vi "Sliding Menu Facade.vi"(0 "Data In":T5, 2 "Display State In":T2={"Numeric"=0.0, "Array of Button References"=[], "Space Between Menu Buttons"=0, "Number of Menu Buttons"=0, "Array of Button Names"=[], "Most Recent Vertical Position"=0, "This VI"=refnum, "Current Action"=enum."Not Moving", "Most Recent Distance Traveled"=0, "Method"=enum."Move Up", "Data In"=0}, 3 "Container State":T6) -> (6 "Data Out":T5, 7 "Display State Out":T2={"Numeric"=0.0, "Array of Button References"=[], "Space Between Menu Buttons"=0, "Number of Menu Buttons"=0, "Array of Button Names"=[], "Most Recent Vertical Position"=0, "This VI"=refnum, "Current Action"=enum."Not Moving", "Most Recent Distance Traveled"=0, "Method"=enum."Move Up", "Data In"=0}, 8 "Action":T1)   [LabVIEW 2011, in "Sliding Menu Library.lvlib" / "Sliding Menu XControl.xctl"]
uses:
  Sliding Menu XControl.xctl
  Sliding Menu Data.ctl
  <vilib>/_xctls/Container State.ctl
  Sliding Menu State.ctl
  Menu Button Library/Menu Button xControl/Menu Button xControl.xctl
  Sliding Menu SubVIs/Sliding Menu Type Definitions/Current User Action.ctl
  Sliding Menu Methods.ctl
  <vilib>/_xctls/Action.ctl
  <vilib>/_xctls/XControlSupport.lvlib
  Sliding Menu Library.lvlib
panel:
  in  "Button 7":bool(xcontrol)
  in  "Button 6":bool(xcontrol)
  in  "Button 5":bool(xcontrol)
  in  "Button 4":bool(xcontrol)
  in  "Button 3":bool(xcontrol)
  in  "Button 2":bool(xcontrol)
  in  "Button 1":bool(xcontrol)
  in  "Button 0":bool(xcontrol)
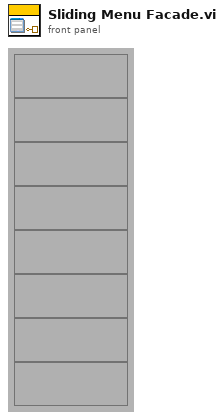
[diagram p1: front panel]
types:
  T1 = typedef "XControlSupport.lvlib/Action.ctl" = cluster{"Data Changed?":bool, "State Changed?":bool, "Action Name":string}
  T2 = typedef "Sliding Menu Library.lvlib/Sliding Menu XControl.xctl/Sliding Menu State.ctl" = cluster{"Numeric":dbl, "Array of Button References":refnum<vi>[], "Space Between Menu Buttons":i32, "Number of Menu Buttons":i32, "Array of Button Names":string[], "Most Recent Vertical Position":i32, "This VI":refnum<vi>, "Current Action":T3, "Most Recent Distance Traveled":i32, "Method":T4, "Data In":T5}
  T3 = typedef "Sliding Menu Library.lvlib/Current User Action.ctl" = enum16{"Not Moving", "Mouse Down", "Mouse Up No Dragging", "Bounce Up Needed", "Bounce Down Needed", "Dragging", "Easing"}
  T4 = typedef "Sliding Menu Methods.ctl" = enum16{"Resize", "Move Up", "Move Down", "Move to 0"}
  T5 = typedef "Sliding Menu Library.lvlib/Sliding Menu XControl.xctl/Sliding Menu Data.ctl" = i32
  T6 = typedef "XControlSupport.lvlib/Container State.ctl" = cluster{"Indicator?":bool, "Run Mode?":bool, " Refnum":refnum<vi>}
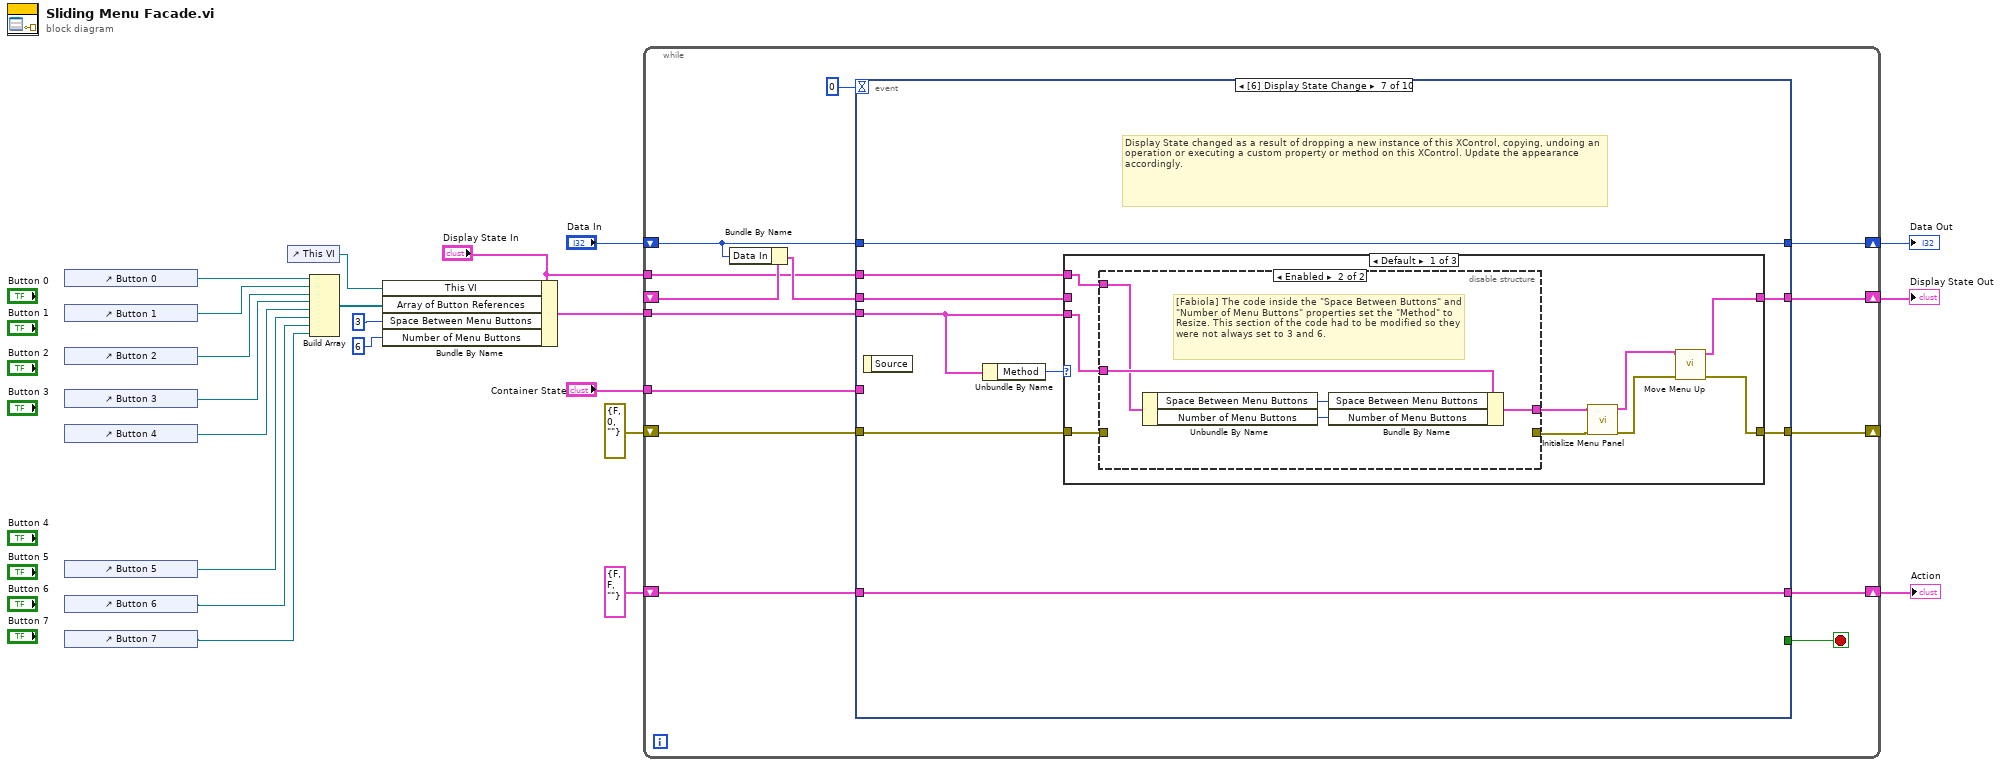
[diagram p0: block diagram]
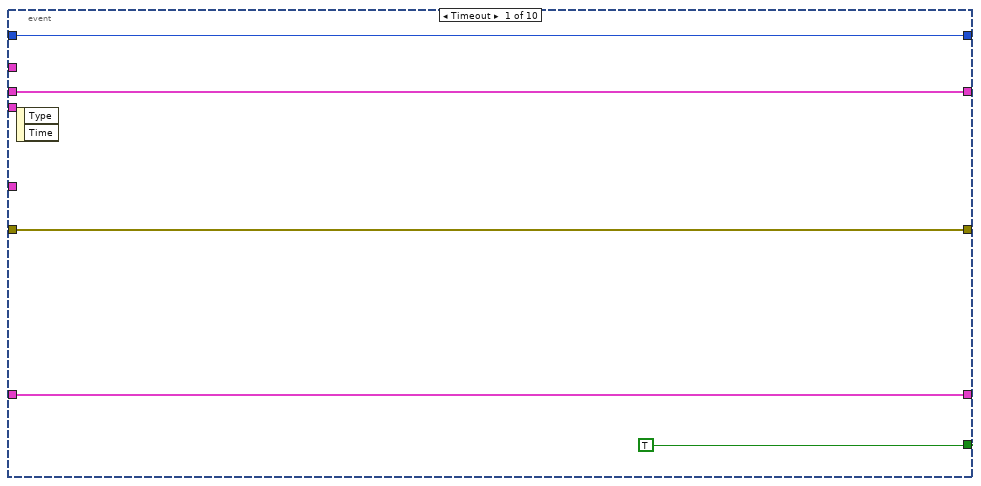
[diagram p2: hidden frame]
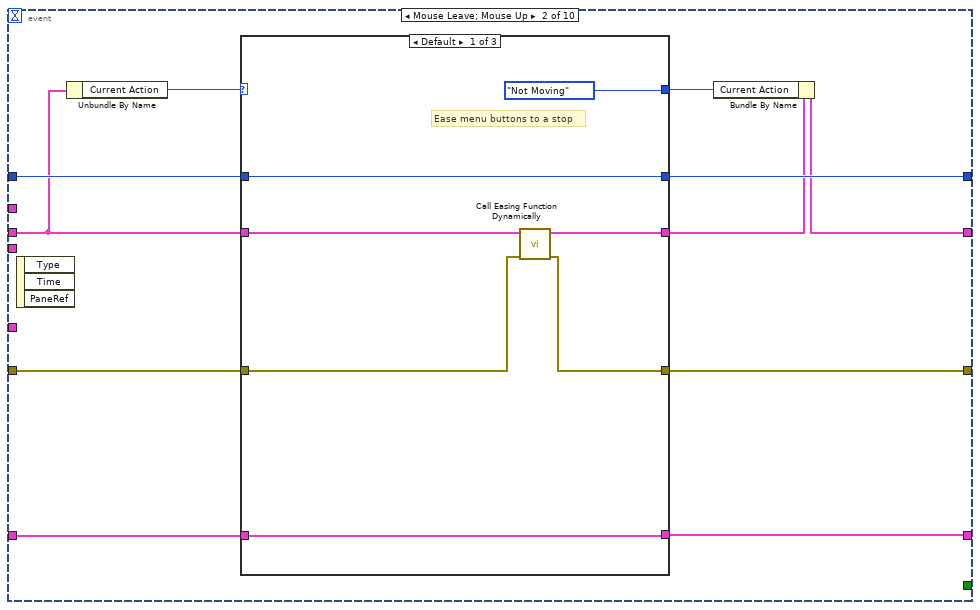
[diagram p3: hidden frame]
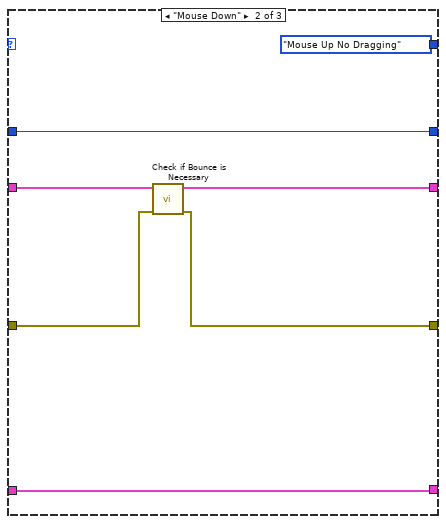
[diagram p4: hidden frame]
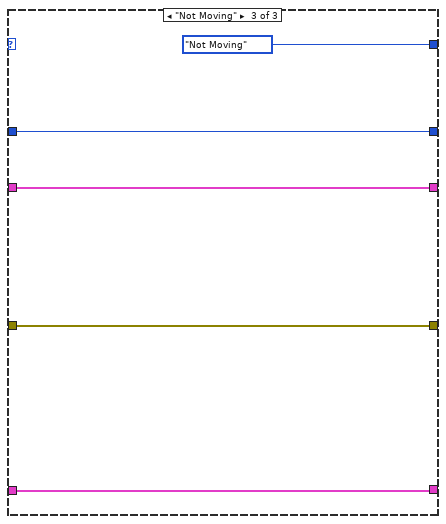
[diagram p5: hidden frame]
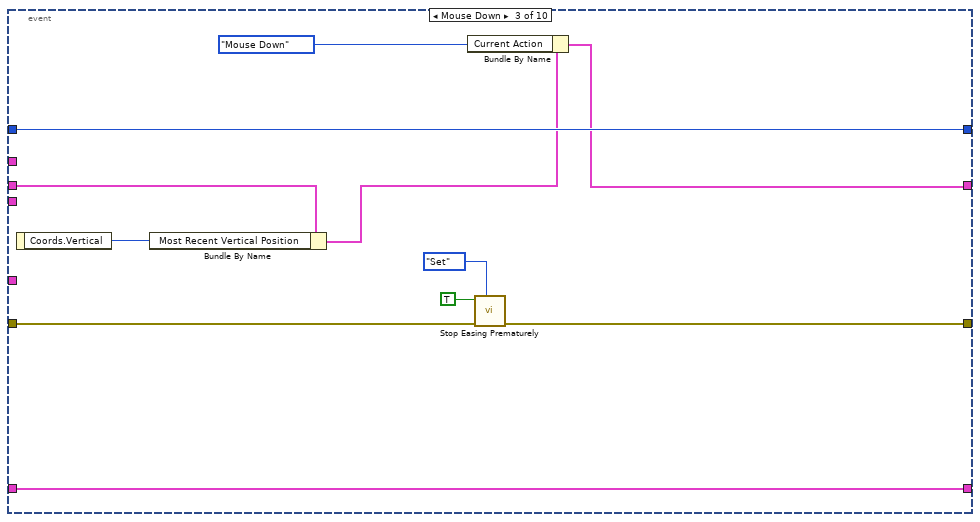
[diagram p6: hidden frame]
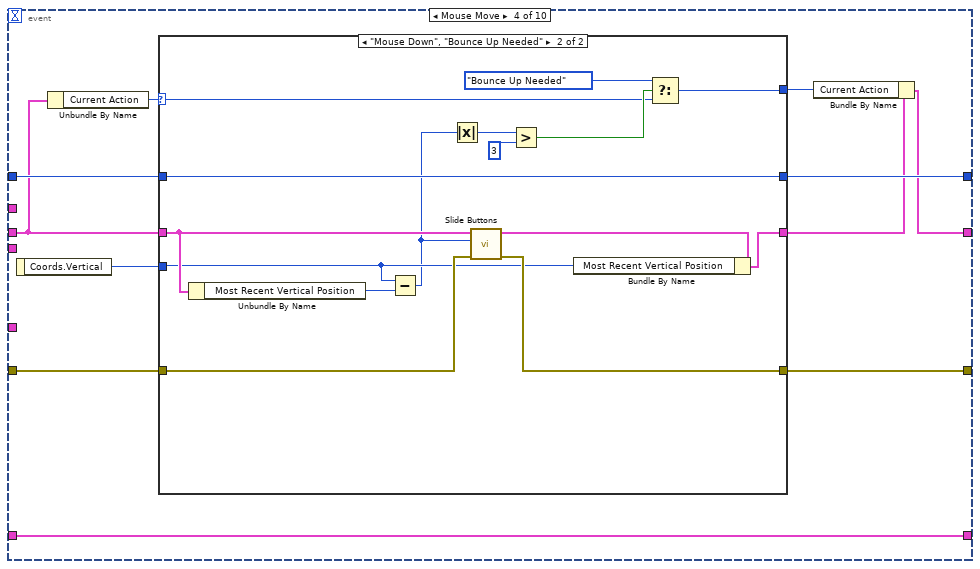
[diagram p7: hidden frame]
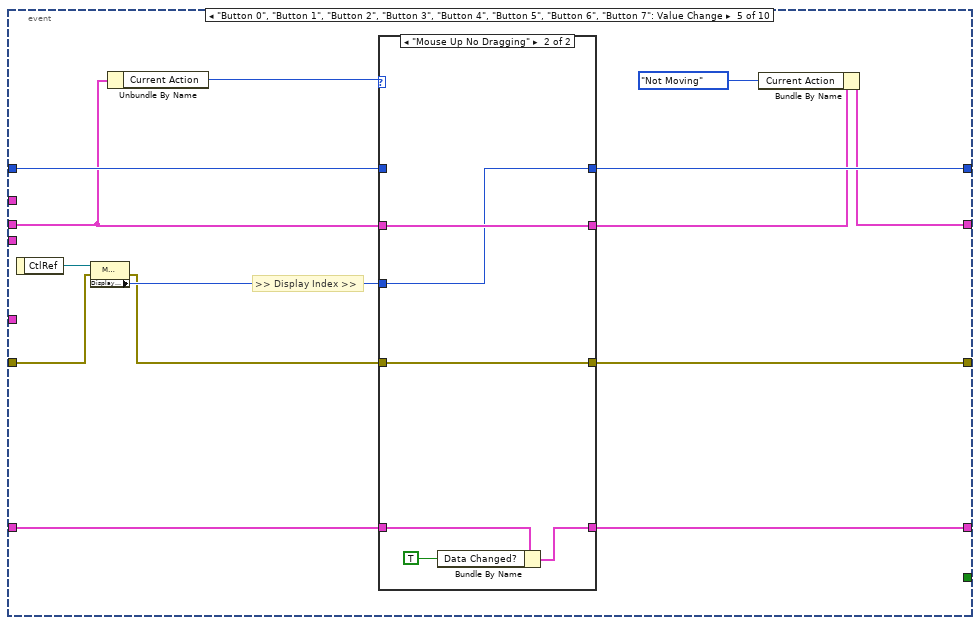
[diagram p9: hidden frame]
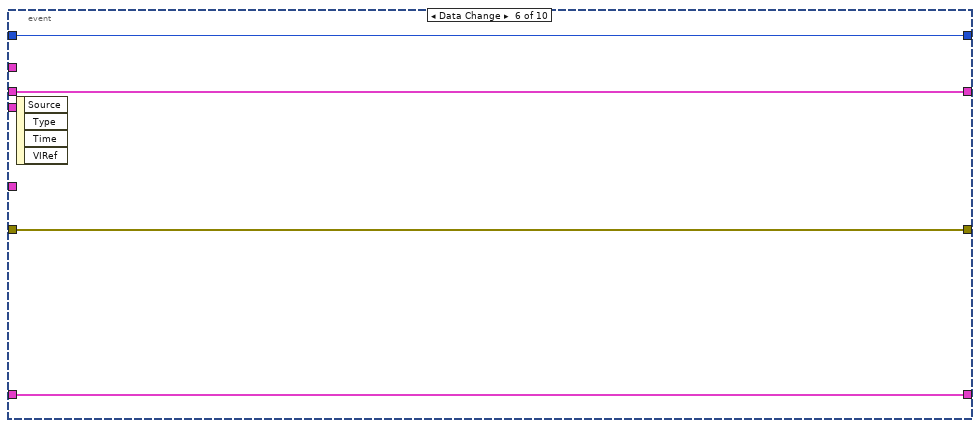
[diagram p11: hidden frame]
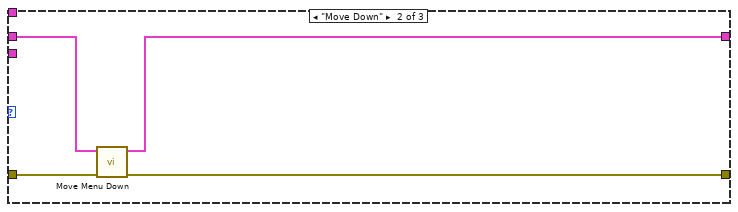
[diagram p13: hidden frame]
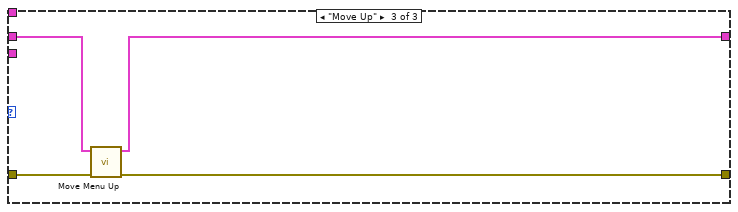
[diagram p14: hidden frame]
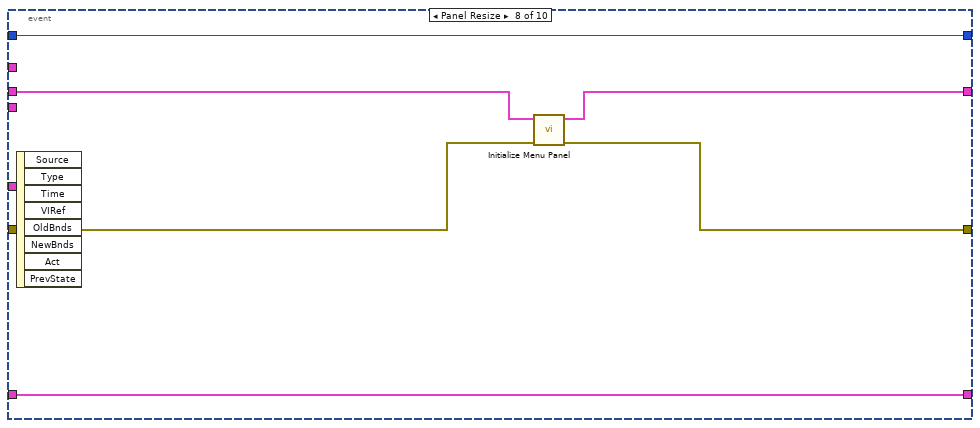
[diagram p15: hidden frame]
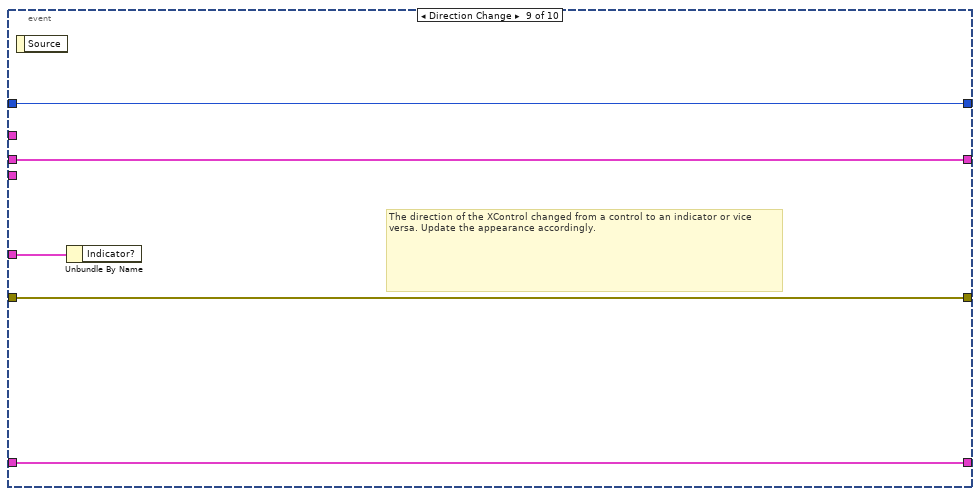
[diagram p16: hidden frame]
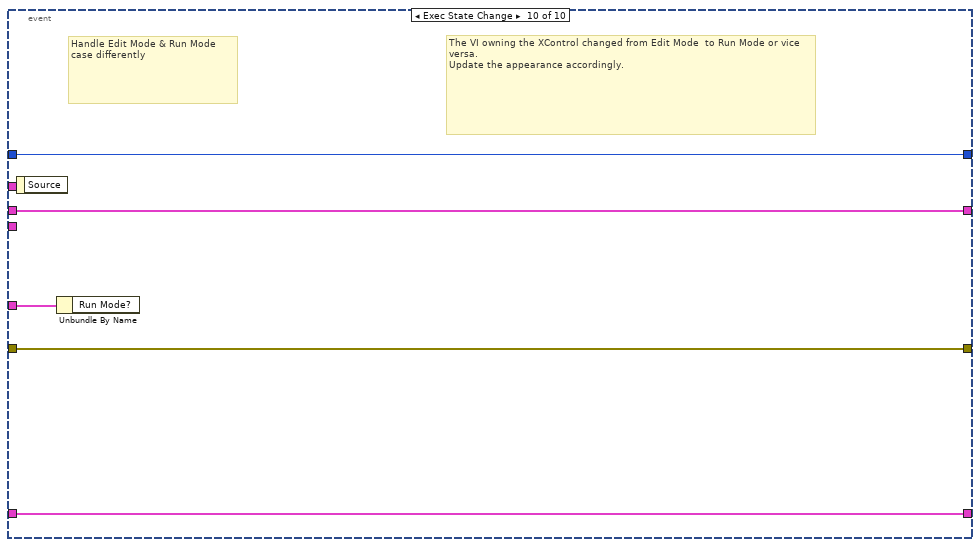
[diagram p17: hidden frame]
diagram:
  n1 = control-ref of="Button 0"() -> (w14:refnum<vi>)
  n2 = control-ref of="Button 1"() -> (w7:refnum<vi>)
  n3 = control-ref of="Button 2"() -> (w8:refnum<vi>)
  n4 = control-ref of="Button 3"() -> (w9:refnum<vi>)
  n5 = control-ref of="Button 4"() -> (w10:refnum<vi>)
  n6 = control-ref of="Button 5"() -> (w11:refnum<vi>)
  n7 = control-ref of="Button 6"() -> (w12:refnum<vi>)
  n8 = control-ref of="Button 7"() -> (w13:refnum<vi>)
  n9 = control-ref of="This VI"() -> (w5:refnum<vi>)
  n10 = Build Array(w14, w7, w8, w9, w10, w11, w12, w13) -> (w6:refnum<vi>[])
  n11 = Bundle By Name(cluster="Display State In", "This VI"=w5, "Array of Button References"=w6, "Space Between Menu Buttons"=3, "Number of Menu Buttons"=6) -> (w4:T2)
  n12 = while {
    shift-right: [w35] -> w19
    shift-left: _ -> [w25]
    tunnel: "Container State" -> [w32]
    shift-right: [w31] -> w21
    shift-left: "Data In" -> [w23]
    shift-right: [w29] -> w18
    shift-left: T1 {"Data Changed?"=FALSE, "State Changed?"=FALSE, "Action Name"=""} ("Action") -> [w30]
    shift-right: [w28] -> _
    shift-left: errorcluster {"status"=FALSE, "code"=0, "source"=""} ("error out") -> [w27]
    tunnel: w4 -> [w26]
    tunnel: "Display State In" -> [w22]
    stop <- w34 stop-if-true
    n13 = Bundle By Name(cluster=w25, "Data In"=w23) -> (w24:T2)
    n14 = event shown="[6] Display State Change" {
      selector: _ -> [_ _ _ _ _ _ _ _ _ _]
      dyn-events: _ -> [_ _ _ _ _ _ _ _ _ _]
      timeout: 0 -> [_ _ _ _ _ _ _ _ _ _]
      tunnel: w24 -> [w38 w45 w79 w86 w115 w138 w141 w176 w182 w187]
      tunnel: [w38 w42 w76 w83 w117 w138 w143 w175 w182 w187] -> w35
      tunnel: [TRUE _ _ _ _ _ _ _ _ _] -> w34
      tunnel: w32 -> [_ _ _ _ _ _ _ _ w183 w188]
      tunnel: w23 -> [w37 w48 w81 w90 w124 w139 w148 w178 w181 w186]
      tunnel: [w37 w49 w81 w91 w125 w139 w148 w178 w181 w186] -> w31
      tunnel: [w39 w46 w80 w92 w112 w137 w147 w177 w180 w185] -> w29
      tunnel: w30 -> [w39 w47 w80 w92 w113 w137 w147 w177 w180 w185]
      tunnel: [w36 w51 w71 w89 w123 w136 w145 w173 w179 w184] -> w28
      tunnel: w27 -> [w36 w50 w72 w88 w120 w136 w146 w174 w179 w184]
      tunnel: w26 -> [_ _ _ _ _ _ w144 _ _ _]
      tunnel: w22 -> [_ _ _ _ _ _ w140 _ _ _]
      event Timeout {
        n15 = event-data() -> ()  [unwired: 1 in, 2 out]
      }
      event Mouse Leave; Mouse Up {
        n16 = event-data() -> ()  [unwired: 1 in, 3 out]
        n17 = Unbundle By Name(w45) -> ("Current Action"=w44:T3)
        n18 = case shown="Default" w44 {
          tunnel: [Current_User_Action."Not Moving" ("Current Action") Current_User_Action."Mouse Up No Dragging" ("Current Action") Current_User_Action."Not Moving" ("Current Action")] -> w41
          tunnel: [w52 w59 w70] -> w51
          tunnel: w50 -> [w55 w60 w70]
          tunnel: [w57 w64 w69] -> w49
          tunnel: w48 -> [w57 w64 w69]
          tunnel: [w53 w61 w68] -> w43
          tunnel: w45 -> [w54 w62 w68]
          tunnel: [w56 w63 w67] -> w46
          tunnel: w47 -> [w56 w63 w67]
          frame Default {
            # "Ease menu buttons to a stop"
            n19 = call "Call Easing Function Dynamically.vi"("error in"=w55, "Display State In"=w54) -> ("error out"=w52:errorcluster, "Display State Out"=w53:T2)  [unwired: 8 in]
          }
          frame "Mouse Down" {
            n20 = call "Check if Bounce is Necessary.vi"("error in"=w60, "Display State In"=w62) -> ("error out"=w59:errorcluster, "Display State Out 2"=w61:T2)  [unwired: 7 in, 1 out]
          }
          frame "Not Moving" {
          }
        }
        n21 = Bundle By Name(cluster=w43, "Current Action"=w41) -> (w42:T2)
      }
      event Mouse Down {
        n22 = event-data() -> ("Coords.Vertical"=w78:i32)  [unwired: 1 in]
        n23 = Bundle By Name(cluster=w79, "Most Recent Vertical Position"=w78) -> (w75:T2)
        n24 = Bundle By Name(cluster=w75, "Current Action"=Current_User_Action."Mouse Down") -> (w76:T2)
        n25 = call "Stop Easing Prematurely.vi"("Set or Get Value"=enum16{"Set", "Get"}."Set", "error in"=w72, "Stop?"=TRUE) -> ("error out"=w71:errorcluster)  [unwired: 7 in, 1 out]
      }
      event Mouse Move {
        n26 = event-data() -> ("Coords.Vertical"=w87:i32)  [unwired: 1 in]
        n27 = Unbundle By Name(w86) -> ("Current Action"=w85:T3)
        n28 = case shown="\"Mouse Down\", \"Bounce Up Needed\"" w85 {
          selector: w85 -> [w93 w99]
          tunnel: [w93 w98] -> w82
          tunnel: [w94 w111] -> w91
          tunnel: w90 -> [w94 w111]
          tunnel: [w95 w104] -> w84
          tunnel: w86 -> [w95 w107]
          tunnel: [w96 w109] -> w89
          tunnel: w88 -> [w96 w110]
          tunnel: w87 -> [_ w106]
          frame Default {
          }
          frame "Mouse Down", "Bounce Up Needed" {
            n29 = Unbundle By Name(w107) -> ("Most Recent Vertical Position"=w108:i32)
            n30 = Subtract(x=w106, y=w108) -> (x-y=w100:i32)
            n31 = Absolute Value(x=w100) -> (abs(x)=w101:i32)
            n32 = call "Slide Buttons.vi"("error in (no error)"=w110, "Distance"=w100, "Display State In"=w107) -> ("error out"=w109:errorcluster, "Display State Out"=w105:T2)  [unwired: 7 in]
            n33 = Greater?(x=w101, y=3) -> (0:w102:bool)
            n34 = Bundle By Name(cluster=w105, "Most Recent Vertical Position"=w106) -> (w104:T2)
            n35 = Select(t=Current_User_Action."Bounce Up Needed", s=w102, f=w99) -> (s? t:f=w98:T3)
          }
        }
        n36 = Bundle By Name(cluster=w84, "Current Action"=w82) -> (w83:T2)
      }
      event "Button 0", "Button 1", "Button 2", "Button 3", "Button 4", "Button 5", "Button 6", "Button 7": Value Change {
        # ">> Display Index >>"
        n37 = event-data() -> ("CtlRef"=w122:refnum<vi>)  [unwired: 1 in]
        n38 = property class="Menu Button xControl (strict)"(reference=w122, error in=w120) -> (error out=w119:errorcluster, "Display Index"=w121:i32)  [unwired: 1 out]
        n39 = Unbundle By Name(w115) -> ("Current Action"=w114:T3)
        n40 = case shown="\"Mouse Up No Dragging\"" w114 {
          tunnel: [w129 w133] -> w125
          tunnel: w124 -> [w129 _]
          tunnel: w115 -> [w128 w135]
          tunnel: [w128 w135] -> w118
          tunnel: [w127 w134] -> w123
          tunnel: w119 -> [w127 w134]
          tunnel: w121 -> [_ w133]
          tunnel: w113 -> [w126 w132]
          tunnel: [w126 w131] -> w112
          frame Default {
          }
          frame "Mouse Up No Dragging" {
            n41 = Bundle By Name(cluster=w132, "Data Changed?"=TRUE) -> (w131:T1)
          }
        }
        n42 = Bundle By Name(cluster=w118, "Current Action"=Current_User_Action."Not Moving") -> (w117:T2)
      }
      event Data Change {
        n43 = event-data() -> ()  [unwired: 1 in, 4 out]
      }
      event Display State Change {
        # "Display State changed as a result of dropping a new instance of this XControl, copying, undoing an operation or executing a custom property or method on this XControl. Update the appearance accordingly."
        n44 = event-data() -> ()  [unwired: 1 in, 1 out]
        n45 = Unbundle By Name(w144) -> ("Method"=w142:T4)
        n46 = case shown="Default" w142 {
          tunnel: w146 -> [w151 w168 w172]
          tunnel: [w154 w167 w171] -> w145
          tunnel: w144 -> [w150 _ _]
          tunnel: [w157 w165 w169] -> w143
          tunnel: w141 -> [_ w166 w170]
          tunnel: w140 -> [w149 _ _]
          frame Default {
            n47 = disable-structure shown="Enabled" {
              disable-tunnel: w150 -> [w159 w163]
              disable-tunnel: [w159 w164] -> w153
              disable-tunnel: [w158 _] -> w152
              disable-tunnel: w151 -> [w158 _]
              disable-tunnel: w149 -> [_ w160]
              frame Disabled {
              }
              frame Enabled {
                # "[Fabiola] The code inside the \"Space Between Buttons\" and \"Number of Menu Buttons\" properties set the \"Method\" to Resize. This section of the code had to be modified so they were not always set to 3 and 6."
                n48 = Unbundle By Name(w160) -> ("Space Between Menu Buttons"=w162:i32, "Number of Menu Buttons"=w161:i32)
                n49 = Bundle By Name(cluster=w163, "Space Between Menu Buttons"=w162, "Number of Menu Buttons"=w161) -> (w164:T2)
              }
            }
            n50 = call "Initialize Menu Panel.vi"("error in"=w152, "Display State In"=w153) -> ("error IO 2"=w155:errorcluster, "Display State Out"=w156:T2)  [unwired: 8 in]
            n51 = call "Move Menu Up.vi"("error in (no error)"=w155, "Display State In"=w156) -> ("error out"=w154:errorcluster, "Display State Out"=w157:T2)  [unwired: 8 in]
          }
          frame "Move Down" {
            n52 = call "Move Menu Down.vi"("error in (no error)"=w168, "Display State In"=w166) -> ("error out"=w167:errorcluster, "Display State Out"=w165:T2)  [unwired: 8 in]
          }
          frame "Move Up" {
            n53 = call "Move Menu Up.vi"("error in (no error)"=w172, "Display State In"=w170) -> ("error out"=w171:errorcluster, "Display State Out"=w169:T2)  [unwired: 8 in]
          }
        }
      }
      event Panel Resize {
        n54 = event-data() -> ()  [unwired: 1 in, 8 out]
        n55 = call "Initialize Menu Panel.vi"("error in"=w174, "Display State In"=w176) -> ("error IO 2"=w173:errorcluster, "Display State Out"=w175:T2)  [unwired: 8 in]
      }
      event Direction Change {
        # "The direction of the XControl changed from a control to an indicator or vice versa. Update the appearance accordingly."
        n56 = event-data() -> ()  [unwired: 1 in, 1 out]
        n57 = Unbundle By Name(w183) -> ()  [unwired: 1 out]
      }
      event Exec State Change {
        # "The VI owning the XControl changed from Edit Mode  to Run Mode or vice versa.\nUpdate the appearance accordingly."
        # "Handle Edit Mode & Run Mode\ncase differently"
        n58 = event-data() -> ()  [unwired: 1 in, 1 out]
        n59 = Unbundle By Name(w188) -> ()  [unwired: 1 out]
      }
    }
  }
  "Display State Out" <- w19
  "Data Out" <- w21
  "Action" <- w18
